vi "TestVirtual1.vi"(0 "reference in":refnum<class "G#BaseClass2_IG#BaseInterface.lvclass">, 5 "error in (no error)":errorcluster) -> (14 "reference out":refnum<class "G#BaseClass2_IG#BaseInterface.lvclass">, 15 "MethodName":string[](array[string]), 19 "error out":errorcluster)   [LabVIEW 2020, in "G#BaseClass2_IG#BaseInterface.lvclass"]
uses:
  G#BaseClass2_IG#BaseInterface.lvclass
  G#BaseClass2.lvclass
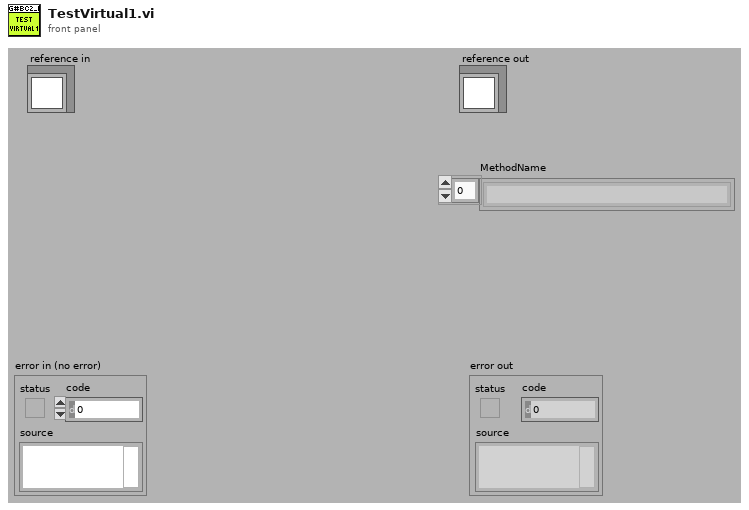
[diagram p1: front panel]
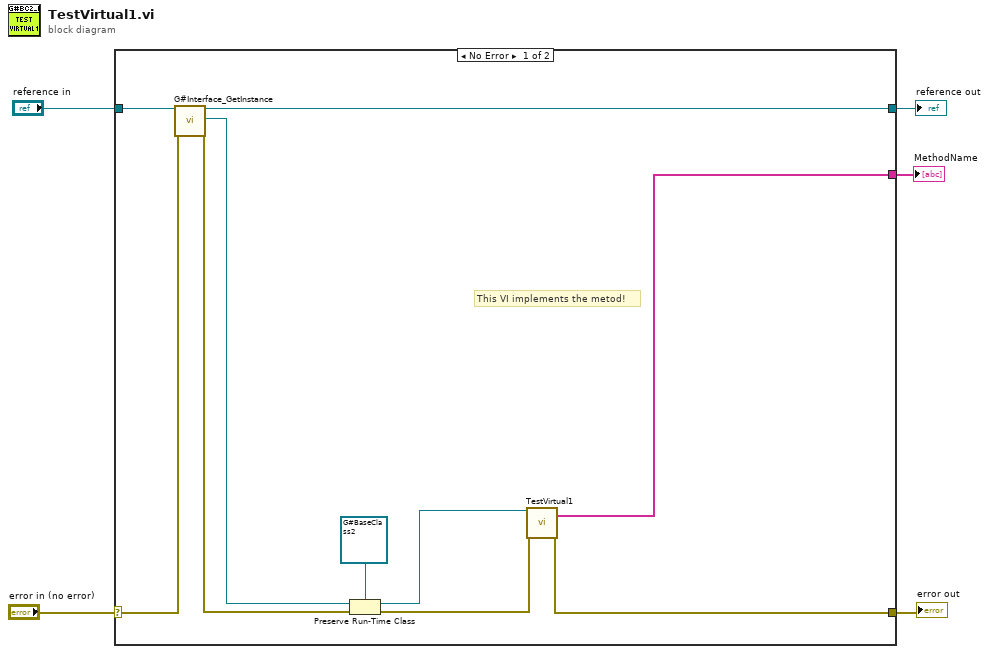
[diagram p0: block diagram]
diagram:
  n1 = case shown="No Error" "error in (no error)" {
    selector: "error in (no error)" -> [w14 w17]
    tunnel: [w8 w17] -> w4
    tunnel: [w11 w16] -> w2
    tunnel: "reference in" -> [w15 w16]
    tunnel: [w6 _] -> w1
    frame No Error {
      # "This VI implements the metod!"
      n2 = call-dynamic "G#Interface_GetInstance.vi"("reference in"=w15, "error in (no error)"=w14) -> ("reference out"=w11:refnum<class "G#BaseClass2_IG#BaseInterface.lvclass">, "G#Object"=w12:refnum<class "G#Object.lvclass">, "error out"=w13:errorcluster)  [unwired: 14 in, 1 out]
      n3 = Preserve Run-Time Class(object in=w12, error in=w13, 2:refnum<class "G#BaseClass2.lvclass"> refnum ("G#BaseClass2.lvclass")) -> (object out=w7:refnum<class "G#BaseClass2.lvclass">, error out=w9:errorcluster)
      n4 = call-dynamic "TestVirtual1.vi"("reference in"=w7, "error in (no error)"=w9) -> ("MethodName"=w6:string[], "error out"=w8:errorcluster)  [unwired: 15 in, 1 out]
    }
    frame Error {
    }
  }
  "error out" <- w4
  "reference out" <- w2
  "MethodName" <- w1
